vi "TPNT_Not_a_Refnum.vi"() -> (0 "Not_an_element_Refnum":T1)   [LabVIEW 2016]
doc: "This VI returns Not A RefNum.\nCopyright 2001 VI Engineering, Inc."
uses:
  TPNT_Refnum.ctl
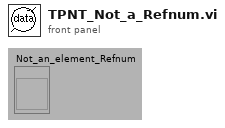
[diagram p1: front panel]
types:
  T1 = typedef "TPNT_Refnum.ctl" = refnum<vi>
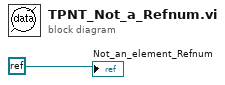
[diagram p0: block diagram]
diagram:
  "Not_an_element_Refnum" <- refnum<k0> refnum
